vi "Tuning.vi"() -> ()   [LabVIEW 2011]
uses:
  point.ctl
panel:
  in  "stop 2":bool
  in  "Y axix PID gains 2":T1={"proportional gain (Kc)"=0.5, "integral time (Ti, min)"=0.01, "derivative time (Td, min)"=0.01}
  in  "X axis PID gains":T1={"proportional gain (Kc)"=0.5, "integral time (Ti, min)"=0.01, "derivative time (Td, min)"=0.01}
  in  "Point":T2
  in  "stop":bool
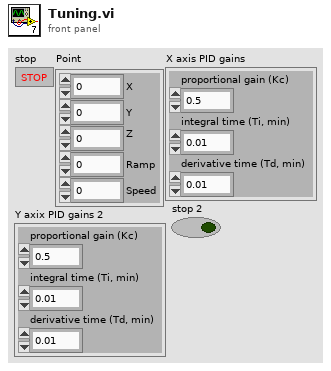
[diagram p1: front panel]
types:
  T1 = cluster{"proportional gain (Kc)":dbl, "integral time (Ti, min)":dbl, "derivative time (Td, min)":dbl}
  T2 = typedef "point.ctl" = cluster{"X":dbl, "Y":dbl, "Z":dbl, "Ramp":dbl, "Speed":dbl}
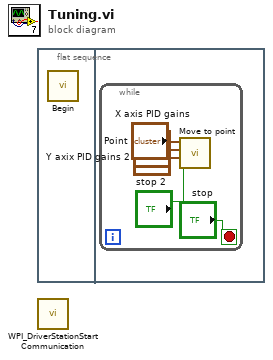
[diagram p0: block diagram]
diagram:
  n1 = flat-sequence {
    frame #0 {
      n2 = call "Begin.vi"() -> ()  [unwired: 11 in, 1 out]
    }
    frame #1 {
      n3 = while {
        stop <- "stop" stop-if-true
        n4 = call "Move to point.vi"(8:"stop 2", 9:"Y axix PID gains 2", 10:"X axis PID gains", "Point"="Point") -> ()  [unwired: 8 in]
      }
    }
  }
  n5 = call <vilib>:"WPI_DriverStationStart Communication.vi"() -> ()  [unwired: 12 in]
